vi "Breaker Reset Delay Expired.vi"(8 "Breaker Reset Ticks":u32=40000000 caption="Tick Count(Ticks)", 9 "Delay (Ticks)":u32, 10 "Reset Breaker":bool, 11 "Reset Switch":bool) -> (2 "Reset Breaker Out":bool, 3 "Timer Running":bool)   [LabVIEW 2018]
doc: "Author: Scott Hannahs <sth@magnet.fsu.edu>\nCopyright 2018 Florida State University, All rights reserved."
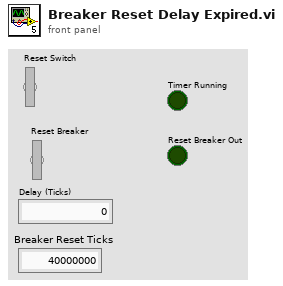
[diagram p1: front panel]
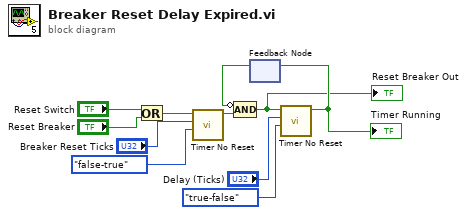
[diagram p0: block diagram]
diagram:
  n1 = Or(x="Reset Switch", y="Reset Breaker") -> (x .or. y?=w4:bool)
  n2 = call "Timer No Reset.vi"("Direction"=enum8{"either", "false-true", "true-false"}."false-true", "Tick Count(Ticks)"="Breaker Reset Ticks", "Start Timer"=w4) -> ("Timer Running"=w3:bool)  [unwired: 8 in]
  n3 = feedback #1() -> (w6:bool)  [unwired: 1 in]
  n4 = Compound Arithmetic op=AND(invert w6, w3) -> (w5:bool)
  "Reset Breaker Out" <- w5
  n5 = call "Timer No Reset.vi"("Direction"=enum8{"either", "false-true", "true-false"}."true-false" ("direction"), "Tick Count(Ticks)"="Delay (Ticks)", "Start Timer"=w5) -> ("Timer Running"=w7:bool)  [unwired: 8 in]
  "Timer Running" <- w7
  n6 = feedback-in #1(w7) -> ()
